vi "CPP-5168PuffReleaseAnalysis.vi"() -> (5 "Plug in titles":string[](array[string]), 7 "Plug in values":string[](array[string]))   [LabVIEW 2011]
uses:
  Controls/Post_Process.ctl
  Globals/Plug_in_data_global.vi
  Globals/Meas_global.vi
  <vilib>/measure/mascope.llb/Transition Measurements 1 chan.vi
  Globals/Dynamic_call_global.ph.vi
  <vilib>/measure/NI_MAPro.lvlib
  <vilib>/Analysis/NI_AALBase.lvlib
panel:
  in  "MedianFilter(points)":i32=3
  in  "PufferCard":tag="PXI1Slot3"
  out "FID2decayConstant":dbl
  out "FID1decayConstant":dbl
  in  "Valvetransition":u16(ring)=1 items=["falling", "rising"]
  out "FFID1 2":cluster{dbl, dbl, dbl[]}[](graph)
  out "Valve":cluster{dbl, dbl, dbl[]}(graph)
  out "ValveShutAt":dbl format="%.2f"
  out "FFID2":T1(graph)
  out "Current Block No":i32
  out "FFID1":cluster{dbl, dbl, dbl[]}[](graph)
  out "SourceOffIndex":i32
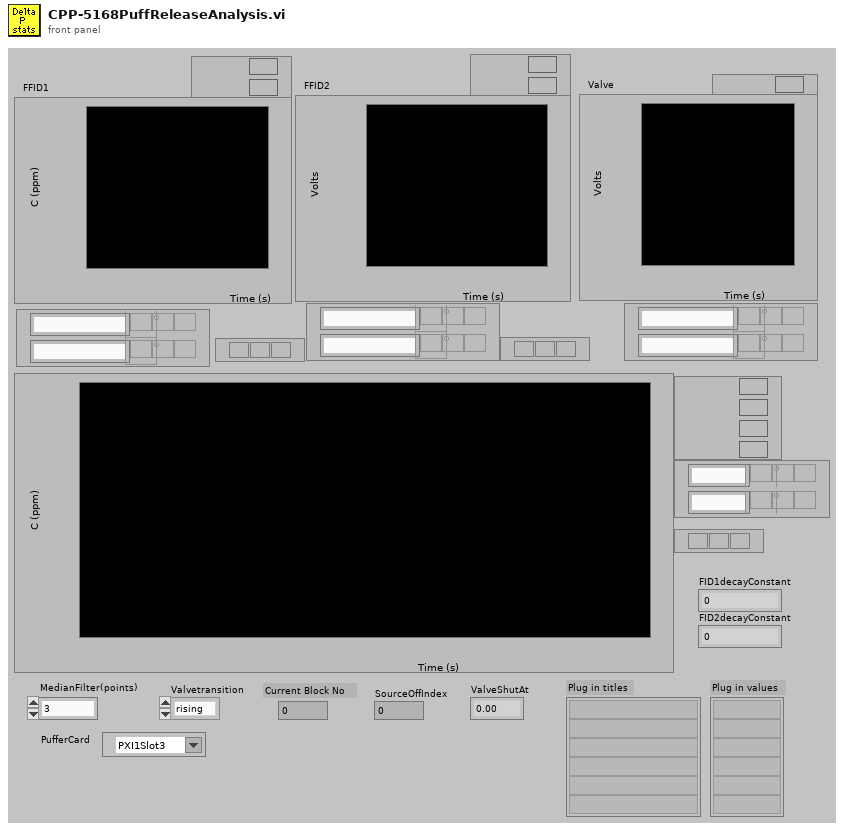
[diagram p1: front panel]
types:
  T1 = cluster{dbl, "SamplingRate":dbl, "Best Exponential Fit":dbl[]}[]
  T2 = enum16{"Save no data", "Save data in new files", "Save data in existing files"}
  T3 = typedef "Post_Process.ctl" = enum16{"Take New Data", "Post Process Raw Data File"}
  T4 = cluster{"start time":dbl, "end time":dbl, "ref levels":cluster{"high ref level":dbl, "mid ref level":dbl, "low ref level":dbl, "ref units":u16}}
  T5 = cluster{dbl, "SamplingRate":dbl, "Best Exponential Fit":dbl[]}
  T6 = cluster{dbl, "SamplingRate":dbl, "Filtered X":dbl[]}[]
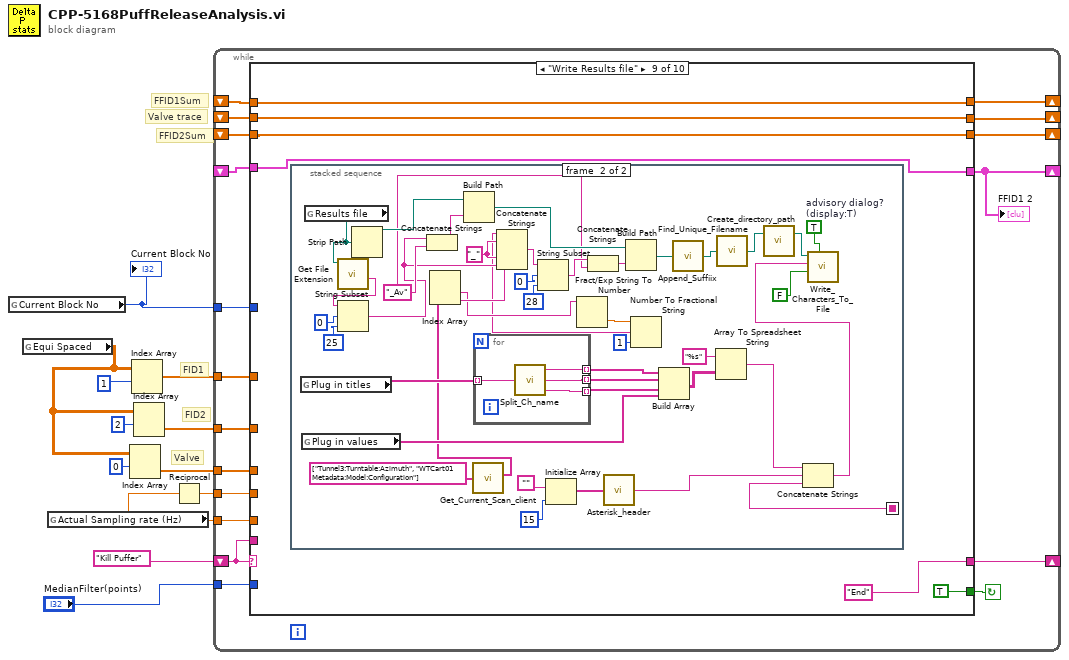
[diagram p0: block diagram]
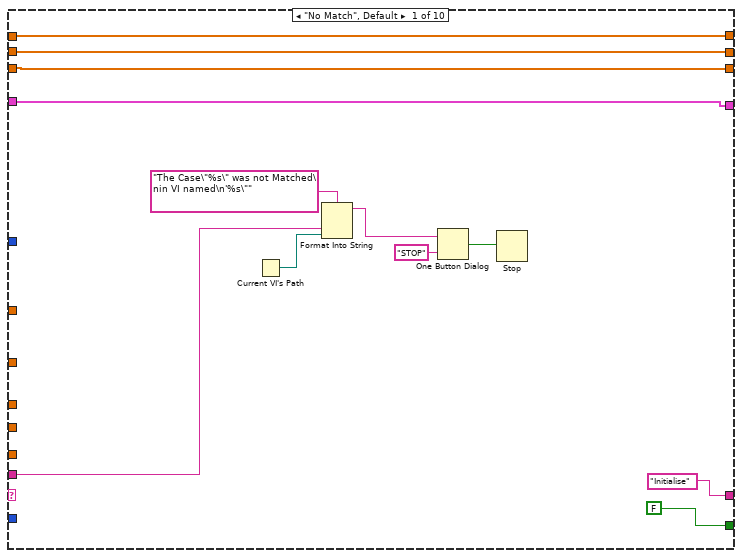
[diagram p2: hidden frame]
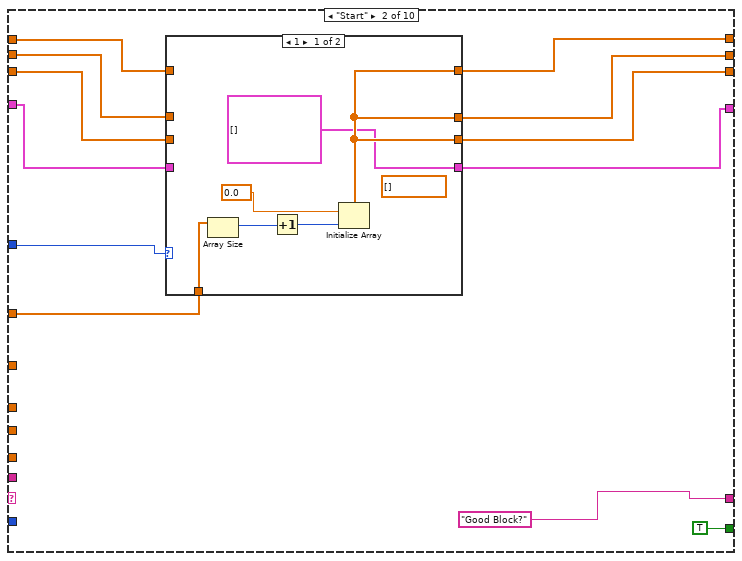
[diagram p3: hidden frame]
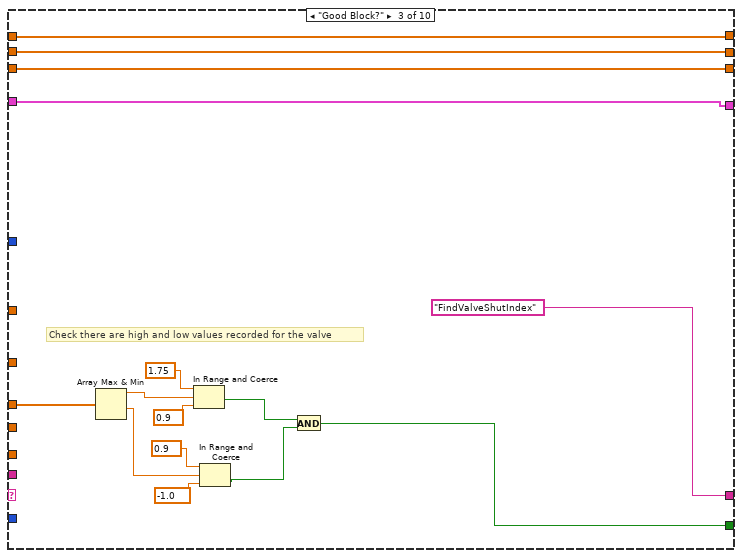
[diagram p5: hidden frame]
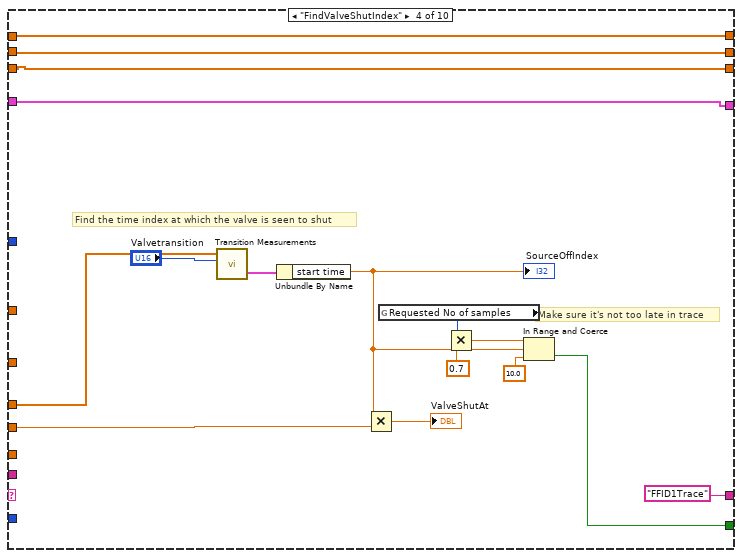
[diagram p6: hidden frame]
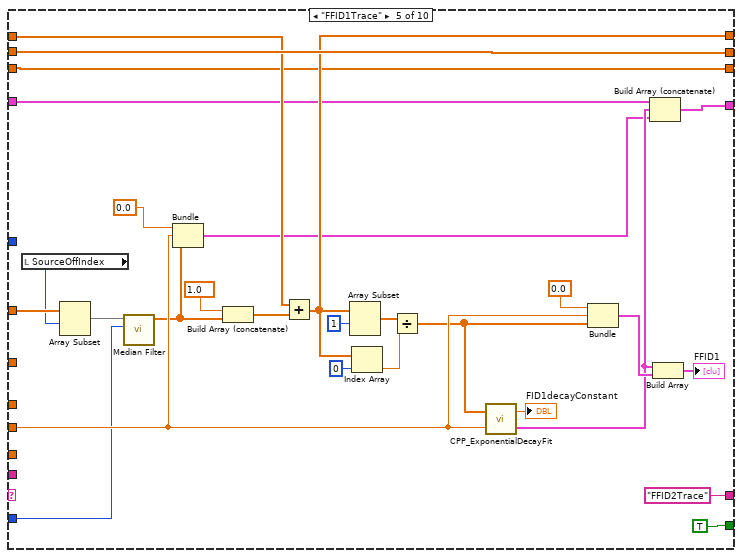
[diagram p7: hidden frame]
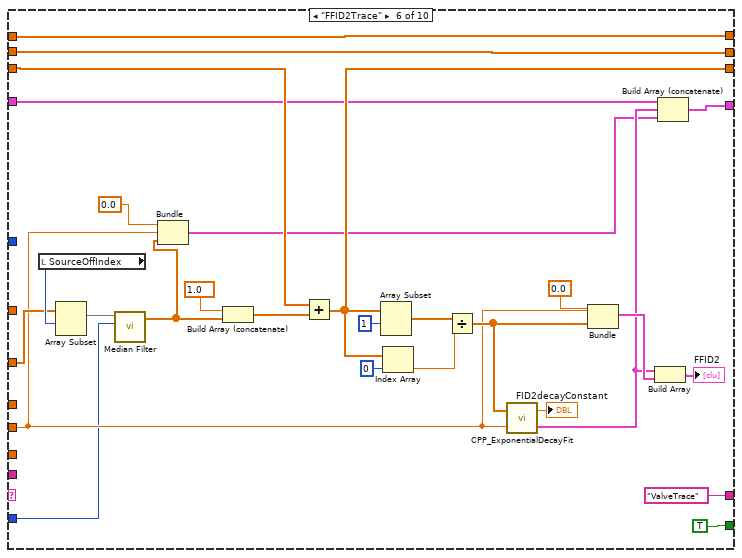
[diagram p8: hidden frame]
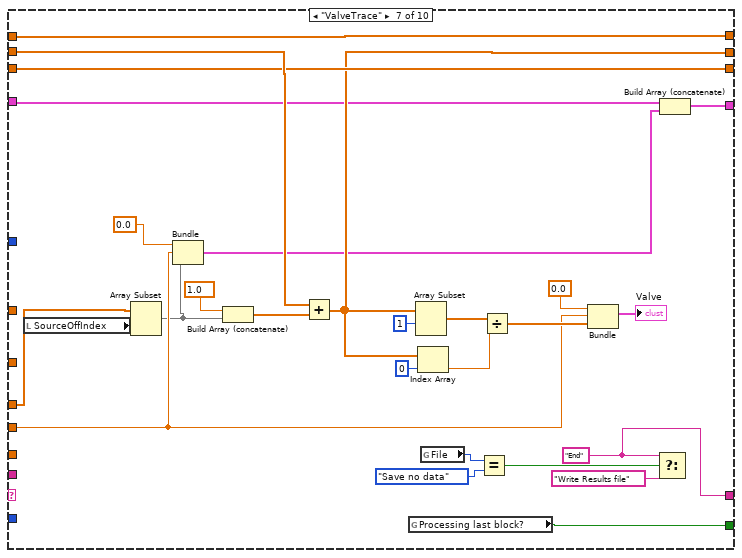
[diagram p9: hidden frame]
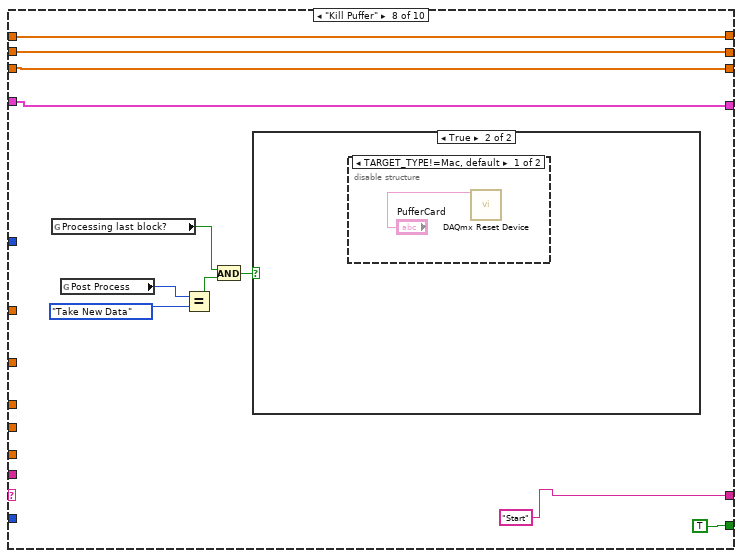
[diagram p10: hidden frame]
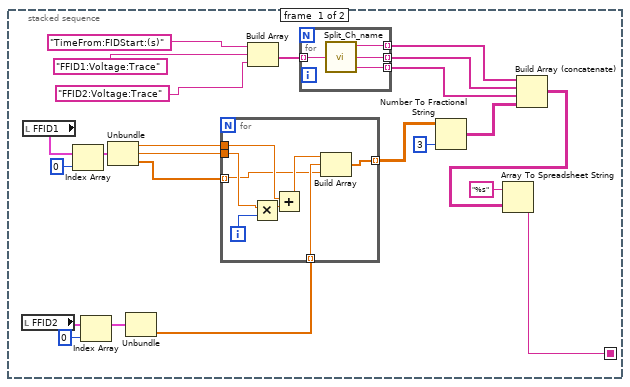
[diagram p13: hidden frame]
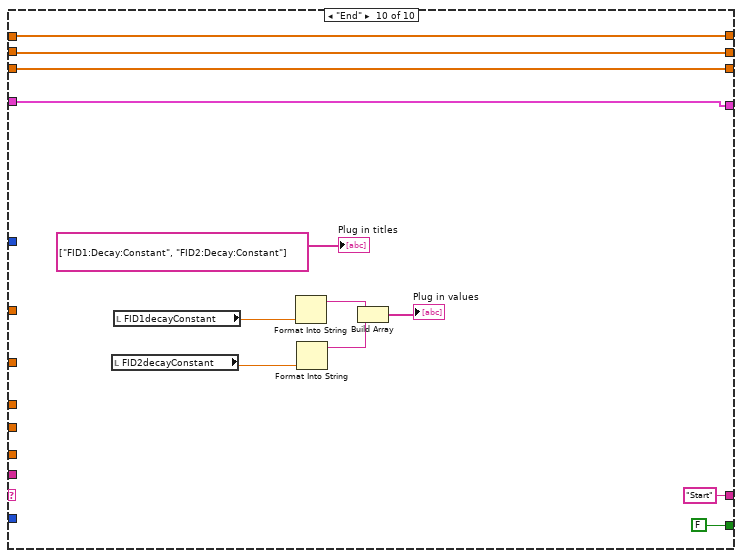
[diagram p14: hidden frame]
diagram:
  # "Valve"
  # "FID2"
  # "FID1"
  # "FFID2Sum"
  # "Valve trace"
  # "FFID1Sum"
  n1 = global read "Meas_global.vi" "Current Block No"() -> (w9:i32)
  "Current Block No" <- w9
  n2 = global read "Plug_in_data_global.vi" "Equi Spaced"() -> (w6:dbl[][])
  n3 = global read "Meas_global.vi" "Actual Sampling rate (Hz)"() -> (w3:dbl)
  n4 = Index Array(array=w6, index (row)=0) -> (element=w5:dbl[])  [unwired: 1 in]
  n5 = Index Array(array=w6, index (row)=1) -> (element=w10:dbl[])  [unwired: 1 in]
  n6 = Index Array(array=w6, index (row)=2) -> (element=w11:dbl[])  [unwired: 1 in]
  n7 = Reciprocal(x=w3) -> (1/x=w2:dbl)
  n8 = while {
    shift-left: "Kill Puffer" -> [w28]
    shift-right: [w29] -> _
    shift-right: [w27] -> _
    shift-left: _ -> [w24]
    shift-right: [w26] -> _
    shift-left: _ -> [w25]
    tunnel: w11 -> [w23]
    tunnel: w10 -> [w22]
    tunnel: w3 -> [w21]
    tunnel: w9 -> [w20]
    shift-right: [w18] -> _
    shift-left: _ -> [w17]
    tunnel: w5 -> [w19]
    tunnel: w2 -> [w16]
    shift-right: [w14] -> _
    shift-left: _ -> [w15]
    tunnel: "MedianFilter(points)" -> [w13]
    stop <- w30 continue-if-true
    n9 = case shown="\"Write Results file\"" w28 {
      tunnel: [FALSE TRUE ("Processing last block?") w74 w84 TRUE ("Processing last block?") TRUE ("Processing last block?") w157 TRUE ("Processing last block?") TRUE ("Processing last block?") FALSE ("Processing last block?")] -> w30
      tunnel: ["Initialise" "Good Block?" "FindValveShutIndex" "FFID1Trace" "FFID2Trace" "ValveTrace" w152 "Start" "End" "Start" ("f")] -> w29
      tunnel: w28 -> [w37 _ _ _ _ _ _ _ _ _]
      tunnel: [w34 w53 w79 w94 w113 w139 w169 w189 w196 w289] -> w27
      tunnel: [w33 w51 w78 w93 w121 w149 w166 w188 w195 w288] -> w26
      tunnel: w25 -> [w33 w50 w78 w93 w121 w149 w168 w188 w195 w288]
      tunnel: w24 -> [w34 w52 w79 w94 w119 w139 w169 w189 w196 w289]
      tunnel: w23 -> [_ _ _ _ _ w140 _ _ _ _]
      tunnel: w22 -> [_ w49 _ _ w120 _ _ _ _ _]
      tunnel: w21 -> [_ _ _ _ _ _ _ _ _ _]
      tunnel: w20 -> [_ w48 _ _ _ _ _ _ _ _]
      tunnel: w19 -> [_ _ w70 w89 _ _ w165 _ _ _]
      tunnel: [w32 w47 w71 w92 w110 w137 w167 w184 w192 w287] -> w18
      tunnel: w17 -> [w32 w46 w71 w92 w110 w138 w167 w184 w192 w287]
      tunnel: w16 -> [_ _ _ w81 w104 w130 w160 _ _ _]
      tunnel: [w31 w44 w65 w80 w108 w136 w164 w180 w191 w284] -> w14
      tunnel: w15 -> [w31 w43 w65 w80 w109 w135 w163 w180 w191 w284]
      tunnel: w13 -> [_ _ _ _ w96 w124 _ _ _ _]
      frame "No Match", Default {
        n10 = Current VI's Path() -> (path=w36:path)
        n11 = Format Into String(format string="The Case\"%s\" was not Matched\nin VI named\n'%s\"" ("Format String"), w37, w36) -> (resulting string=w40:string)  [unwired: 2 in, 1 out]
        n12 = One Button Dialog(message=w40, button name ("OK")="STOP") -> (true=w38:bool)
        n13 = Stop(stop? (T)=w38) -> ()
      }
      frame "Start" {
        n14 = case shown="1" w48 {
          tunnel: [w57 w64] -> w53
          tunnel: w52 -> [_ w64]
          tunnel: [w57 w63] -> w51
          tunnel: w50 -> [_ w63]
          tunnel: w49 -> [w60 _]
          tunnel: [w57 w62] -> w47
          tunnel: w46 -> [_ w62]
          tunnel: [cluster{dbl, dbl, dbl[]}[] [] w61] -> w44
          tunnel: w43 -> [_ w61]
          frame 1 {
            (unwired) dbl[] []
            n15 = Array Size(array=w60) -> (size(s)=w59:i32)
            n16 = Increment(x=w59) -> (x+1=w56:i32)
            n17 = Initialize Array(0.0 ("element"), w56) -> (w57:dbl[])
          }
          frame 2, Default {
          }
        }
      }
      frame "Good Block?" {
        # "Check there are high and low values recorded for the valve"
        n18 = Array Max & Min(array=w70) -> (max value=w73:dbl, min value=w67:dbl)  [unwired: 2 out]
        n19 = In Range and Coerce(upper limit=1.75, x=w73, lower limit=0.9 ("y")) -> (In Range?=w75:bool)  [unwired: 1 out]
        n20 = In Range and Coerce(upper limit=0.9, x=w67, lower limit=-1.0 ("y")) -> (In Range?=w66:bool)  [unwired: 1 out]
        n21 = And(x=w75, y=w66) -> (x .and. y?=w74:bool)
      }
      frame "FindValveShutIndex" {
        # "Make sure it's not too late in trace"
        # "Find the time index at which the valve is seen to shut"
        n22 = call-poly <vilib>:"Transition Measurements.vi"("polarity (rising)"="Valvetransition", "signal in"=w89) -> ("measurement info"=w90:T4)  [unwired: 4 in, 5 out]
        n23 = Unbundle By Name(w90) -> ("start time"=w83:dbl)
        "SourceOffIndex" <- w83
        n24 = Multiply(x=w83, y=w81) -> (x*y=→"ValveShutAt":dbl)
        n25 = global read "Meas_global.vi" "Requested No of samples"() -> (w88:i32)
        n26 = Multiply(x=w88, y=0.7 ("lower limit")) -> (x*y=w86:dbl)
        n27 = In Range and Coerce(upper limit=w86, x=w83, lower limit=10.0) -> (In Range?=w84:bool)  [unwired: 1 out]
      }
      frame "FFID1Trace" {
        n28 = local read "SourceOffIndex"() -> (w116:i32)
        n29 = Array Subset(array=w120, index=w116) -> (w97:dbl[])  [unwired: 1 in]
        n30 = call <vilib>:"Median Filter.vi"("left rank"=w96, "X"=w97) -> ("Filtered X"=w98:dbl[])  [unwired: 8 in, 1 out]
        n31 = Bundle(0.0, w104, "Filtered X"=w98) -> (w100:cluster{dbl, dbl, "Filtered X":dbl[]})  [unwired: 1 out]
        n32 = Build Array (concatenate)(1.0, w98) -> (w117:dbl[])
        n33 = Add(x=w119, y=w117) -> (x+y=w113:dbl[])
        n34 = Array Subset(array=w113, index=1) -> (w112:dbl[])  [unwired: 1 in]
        n35 = Index Array(array=w113, index=0) -> (element=w111:dbl)
        n36 = Divide(x=w112, y=w111) -> (x/y=w99:dbl[])
        n37 = call "CPP_ExponentialDecayFit.vi"("SamplingRate"=w104, "DecayData"=w99) -> ("graphCluster"=w101:T5, "decayConstant"=→"FID1decayConstant":dbl)
        n38 = Bundle(0.0, w104, w99) -> (w102:cluster{dbl, dbl, dbl[]})  [unwired: 1 out]
        n39 = Build Array (concatenate)(w109, w101, w100) -> (w108:T6)
        n40 = Build Array(w101, w102) -> (→"FFID1":T1)
      }
      frame "FFID2Trace" {
        n41 = local read "SourceOffIndex"() -> (w146:i32)
        n42 = Array Subset(array=w140, index=w146) -> (w125:dbl[])  [unwired: 1 in]
        n43 = call <vilib>:"Median Filter.vi"("left rank"=w124, "X"=w125) -> ("Filtered X"=w126:dbl[])  [unwired: 8 in, 1 out]
        n44 = Bundle(0.0, w130, "Filtered X"=w126) -> (w127:cluster{dbl, dbl, "Filtered X":dbl[]})  [unwired: 1 out]
        n45 = Build Array (concatenate)(1.0, w126) -> (w147:dbl[])
        n46 = Add(x=w138, y=w147) -> (x+y=w137:dbl[])
        n47 = Array Subset(array=w137, index=1) -> (w142:dbl[])  [unwired: 1 in]
        n48 = Index Array(array=w137, index=0) -> (element=w141:dbl)
        n49 = Divide(x=w142, y=w141) -> (x/y=w131:dbl[])
        n50 = call "CPP_ExponentialDecayFit.vi"("SamplingRate"=w130, "DecayData"=w131) -> ("graphCluster"=w128:T5, "decayConstant"=→"FID2decayConstant":dbl)
        n51 = Bundle(0.0, w130, w131) -> (w129:cluster{dbl, dbl, dbl[]})  [unwired: 1 out]
        n52 = Build Array(w128, w129) -> (→"FFID2":T1)
        n53 = Build Array (concatenate)(w135, w128, w127) -> (w136:T6)
      }
      frame "ValveTrace" {
        w152 = "End"
        n54 = local read "SourceOffIndex"() -> (w176:i32)
        n55 = Array Subset(array=w165, index=w176) -> (w159:dbl[])  [unwired: 1 in]
        n56 = Bundle(0.0, w160, w159) -> (w158:cluster{dbl, dbl, dbl[]})  [unwired: 1 out]
        n57 = Build Array (concatenate)(1.0, w159) -> (w177:dbl[])
        n58 = Add(x=w168, y=w177) -> (x+y=w166:dbl[])
        n59 = global read "Meas_global.vi" "Processing last block?"() -> (w157:bool)
        n60 = Array Subset(array=w166, index=1) -> (w171:dbl[])  [unwired: 1 in]
        n61 = Index Array(array=w166, index=0) -> (element=w170:dbl)
        n62 = global read "Meas_global.vi" "File"() -> (w156:T2)
        n63 = Equal?(x=w156, y=T2."Save no data" ("File")) -> (x = y?=w153:bool)
        n64 = Divide(x=w171, y=w170) -> (x/y=w175:dbl[])
        n65 = Bundle(0.0, w160, w175) -> (→"Valve":cluster{dbl, dbl, dbl[]})  [unwired: 1 out]
        n66 = Select(t=w152, s=w153, f="Write Results file") -> ()  [unwired: 1 out]
        n67 = Build Array (concatenate)(w163, w158) -> (w164:T6)
      }
      frame "Kill Puffer" {
        n68 = global read "Meas_global.vi" "Processing last block?"() -> (w183:bool)
        n69 = global read "Meas_global.vi" "Post Process"() -> (w186:T3)
        n70 = Equal?(x=w186, y=Post_Process."Take New Data" ("Post Process")) -> (x = y?=w182:bool)
        n71 = And(x=w183, y=w182) -> (x .and. y?=w181:bool)
        n72 = case shown="True" w181 {
          frame False {
          }
          frame True {
            n73 = disable-structure shown="TARGET_TYPE!=Mac, default" {
              frame condition #0 {
                n74 = call <vilib>:"DAQmx Reset Device.vi"("device in"="PufferCard") -> ()  [unwired: 14 in, 1 out]
              }
              frame condition #1 (active) {
              }
            }
          }
        }
      }
      frame "Write Results file" {
        n75 = stacked-sequence {
          seq-local: [w209 _] -> [_ w259]
          frame #0 {
            n76 = local read "FFID2"() -> (w208:T1)
            n77 = local read "FFID1"() -> (w219:cluster{dbl, dbl, dbl[]}[])
            n78 = Index Array(array=w219, index=0) -> (element=w200:cluster{dbl, dbl, dbl[]})
            n79 = Index Array(array=w208, index=0) -> (element=w198:T5)
            n80 = Unbundle(w200) -> (w217:dbl, w218:dbl, w216:dbl[])
            n81 = Unbundle(w198) -> ("Best Exponential Fit"=w207:dbl[])  [unwired: 2 out]
            n82 = for {
              tunnel: w218 -> [w230]
              tunnel: w217 -> [w229]
              tunnel: w216 -> [w224] mode=indexing
              tunnel: [w227] -> w214 mode=indexing
              tunnel: w207 -> [w225] mode=indexing
              i -> [w231]
              n83 = Multiply(x=w230, y=w231) -> (x*y=w228:dbl)
              n84 = Add(x=w229, y=w228) -> (x+y=w226:dbl)
              n85 = Build Array(w226, w225, w224) -> (w227:dbl[])
            }
            n86 = Build Array("TimeFrom:FIDStart:(s)", "FFID1:Voltage:Trace", "FFID2:Voltage:Trace") -> (w204:string[])
            n87 = for {
              tunnel: w204 -> [w223] mode=indexing
              tunnel: [w222] -> w203 mode=indexing
              tunnel: [w221] -> w202 mode=indexing
              tunnel: [w220] -> w201 mode=indexing
              n88 = call "Split_Ch_name.vi"("Ch name"=w223) -> ("Top level"=w222:string, "Middle"=w221:string, "Low level"=w220:string)
            }
            n89 = Number To Fractional String(number=w214, precision (6)=i16 3) -> (F-format string=w213:string[][])  [unwired: 2 out]
            n90 = Build Array (concatenate)(w203, w202, w201, w213) -> (w211:string[][])
            n91 = Array To Spreadsheet String(array=w211, 3:"%s" ("format string")) -> (spreadsheet string=w209:string)  [unwired: 1 out]
          }
          frame #1 {
            w247 = "_" ("string")
            w273 = TRUE  # advisory dialog? (display:T)
            w243 = "_Av" ("string")
            n92 = global read "Dynamic_call_global.ph.vi" "Plug in titles"() -> (w271:string[])
            n93 = global read "Dynamic_call_global.ph.vi" "Plug in values"() -> (w267:string[])
            n94 = global read "Meas_global.vi" "Results file"() -> (w253:path)
            n95 = call <vilib>:"Get File Extension.vi"("file"=w253) -> ("filename without extension"=w239:string)  [unwired: 7 in, 3 out]
            n96 = String Subset(string=w239, offset (0)=0, length (rest)=25 ("length (rest)")) -> (substring=w238:string)
            n97 = Strip Path(path=w253) -> (stripped path=w252:path)  [unwired: 1 out]
            n98 = Concatenate Strings(w238, w243) -> (w250:string)
            n99 = Build Path(base path=w252, name or relative path=w250) -> (appended path=w251:path)
            n100 = call "Get_Current_Scan_client.vi"("ADAM Ch Names"=string[] ["Tunnel3:Turntable:Azimuth", "WTCart01 Metadata:Model:Configuration"]) -> ("String values"=w248:string[])  [unwired: 1 in, 2 out]
            n101 = Index Array(array=w248) -> (element #1=w235:string, element #2=w246:string)  [unwired: 2 in]
            n102 = for {
              tunnel: w271 -> [w277] mode=indexing
              tunnel: [w276] -> w270 mode=indexing
              tunnel: [w275] -> w269 mode=indexing
              tunnel: [w274] -> w268 mode=indexing
              n103 = call "Split_Ch_name.vi"("Ch name"=w277) -> ("Top level"=w276:string, "Middle"=w275:string, "Low level"=w274:string)
            }
            n104 = Initialize Array("", 15) -> (w264:string[])
            n105 = Fract/Exp String To Number(string=w235) -> (number=w234:dbl)  [unwired: 3 in, 1 out]
            n106 = call "Asterisk_header.vi"("Channel names"=w264) -> ("Header string"=w260:string)
            n107 = Number To Fractional String(number=w234, precision (6)=i16 1) -> (F-format string=w232:string)  [unwired: 2 in]
            n108 = Concatenate Strings(w232, w247, w246, w247, w238) -> (w245:string)
            n109 = String Subset(string=w245, offset (0)=0, length (rest)=28 ("length (rest)")) -> (substring=w244:string)
            n110 = Concatenate Strings(w244, w243) -> (w242:string)
            n111 = Build Path(base path=w251, name or relative path=w242) -> (appended path=w255:path)
            n112 = Build Array(w270, w269, w268, w267) -> (w265:string[][])
            n113 = call "Append_Suffiix.vi"("Results file"=w255) -> ("appended path"=w254:path)
            n114 = Array To Spreadsheet String(array=w265, 3:"%s" ("format string")) -> (spreadsheet string=w261:string)  [unwired: 1 out]
            n115 = call "Find_Unique_Filename.vi"("Path In"=w254) -> ("Unique Path Out"=w237:path)  [unwired: 1 in, 1 out]
            n116 = call "Create_directory_path.vi"("Path name"=w237) -> ("Path name Out"=w236:path)  [unwired: 1 in, 1 out]
            n117 = Concatenate Strings(w261, w260, w259) -> (w258:string)
            n118 = call "Write_Characters_To_File.vi"("file path (dialog if empty)"=w236, "advisory dialog? (display:T)"=w273, "character string"=w258, "append to file? (new file:F)"=FALSE) -> ()  [unwired: 1 in, 4 out]
          }
        }
      }
      frame "End" {
        n119 = local read "FID2decayConstant"() -> (w280:dbl)
        n120 = local read "FID1decayConstant"() -> (w282:dbl)
        n121 = Format Into String(w282) -> (resulting string=w281:string)  [unwired: 3 in, 1 out]
        n122 = Format Into String(w280) -> (resulting string=w279:string)  [unwired: 3 in, 1 out]
        n123 = Build Array(w281, w279) -> (→"Plug in values":string[])
        "Plug in titles" <- string[] ["FID1:Decay:Constant", "FID2:Decay:Constant"] ("Plug in titles")
      }
    }
    "FFID1 2" <- w14
  }
